vi "RSNRPZshowMeasurement.vi"(8 "error in (no error)":errorcluster, 9 "Rolling average : 3":refnum<vi>, 10 "Measurement":dbl format="%.3p", 11 "RSNPRZgraph 2":refnum<vi>) -> (0 "error out":errorcluster, 3 "power out":dbl)   [LabVIEW 2019]
uses:
  <vilib>/ptbypt/NI_PtbyPt.lvlib
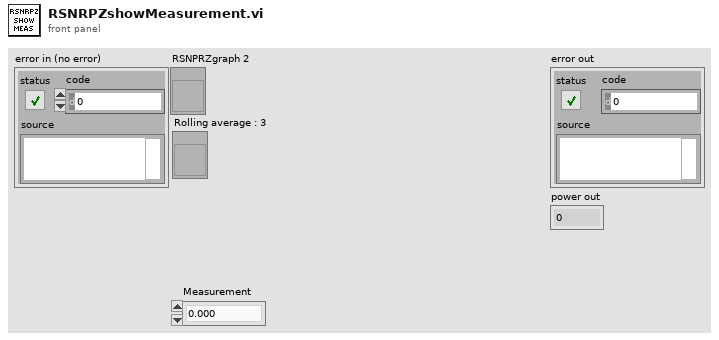
[diagram p1: front panel]
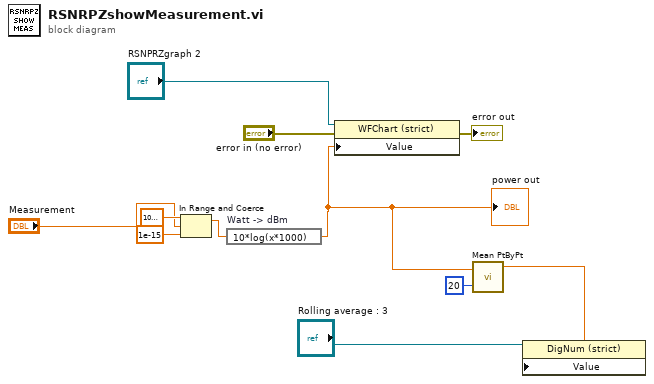
[diagram p0: block diagram]
diagram:
  n1 = In Range and Coerce(upper limit=1000000.0 ("Scope Time (0.01 s)"), x="Measurement", lower limit=1e-15 ("Scope Time (0.01 s)")) -> (coerced(x)=w6:dbl)  [unwired: 1 out]
  n2 = expression code="10*log(x*1000)" "Watt -> dBm"(w6) -> (w3:dbl)
  "power out" <- w3
  n3 = property class="WFChart (strict)"(reference="RSNPRZgraph 2", error in="error in (no error)", "Value"=w3) -> (error out=→"error out":errorcluster)  [unwired: 1 out]
  n4 = call <vilib>:"Mean PtByPt.vi"("x"=w3, "sample length"=20) -> ("mean"=w1:dbl)  [unwired: 2 in, 1 out]
  n5 = property class="DigNum (strict)"(reference="Rolling average : 3", "Value"=w1) -> ()  [unwired: 1 in, 2 out]
